vi "AcquiringASignal.vi"() -> ()   [LabVIEW 2025]
panel:
  in  "Knob":dbl(knob) scale=0.0..10.0
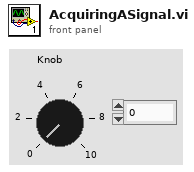
[diagram p1: front panel]
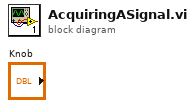
[diagram p0: block diagram]
diagram:
